vi "Save Correction.vi"() -> ()   [LabVIEW 2017]
uses:
  Globals.vi
panel:
  out "Boolean":bool=TRUE
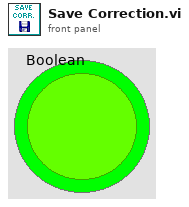
[diagram p1: front panel]
types:
  T1 = cluster{"x shift":dbl, "y shift":dbl, "z shift":dbl, "Theta x":dbl, "Theta y":dbl}
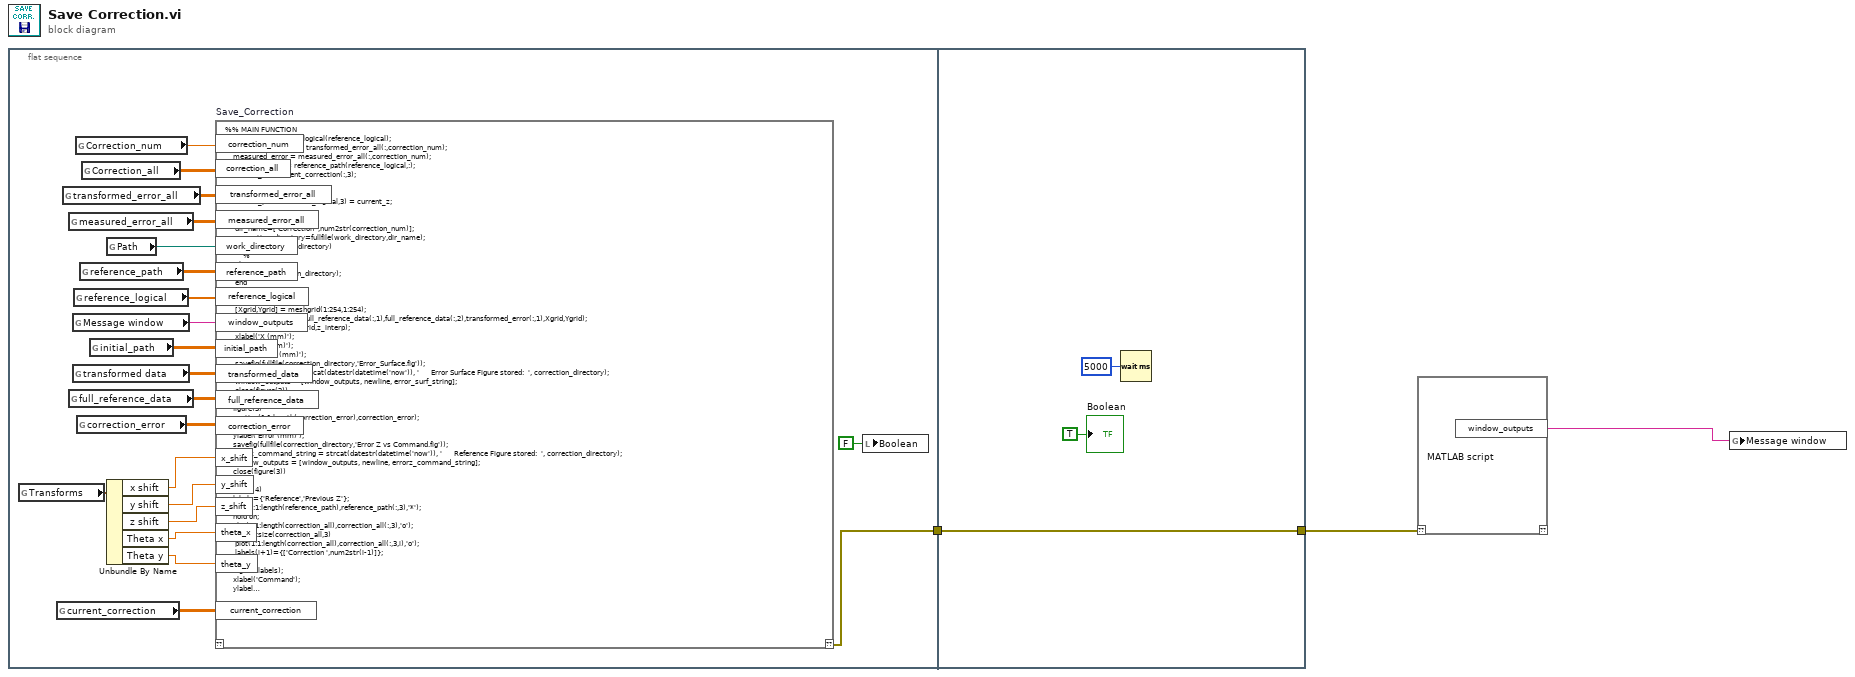
[diagram p0: block diagram]
diagram:
  n1 = flat-sequence {
    tunnel: [w5] -> w1
    tunnel: [w27] -> w2
    tunnel: w1 -> [w27]
    frame #0 {
      n2 = global read "Globals.vi" "Transforms"() -> (w12:T1)
      n3 = global read "Globals.vi" "current_correction"() -> (w6:dbl[][])
      n4 = global read "Globals.vi" "transformed_error_all"() -> (w15:dbl[][])
      n5 = global read "Globals.vi" "measured_error_all"() -> (w16:dbl[][])
      n6 = global read "Globals.vi" "full_reference_data"() -> (w23:dbl[][])
      n7 = global read "Globals.vi" "Message window"() -> (w20:string)
      n8 = global read "Globals.vi" "transformed data"() -> (w22:dbl[][])
      n9 = global read "Globals.vi" "reference_logical"() -> (w19:dbl[])
      n10 = global read "Globals.vi" "Correction_num"() -> (w13:dbl)
      n11 = global read "Globals.vi" "correction_error"() -> (w24:dbl[][])
      n12 = global read "Globals.vi" "reference_path"() -> (w18:dbl[][])
      n13 = global read "Globals.vi" "Correction_all"() -> (w14:dbl[][])
      n14 = global read "Globals.vi" "initial_path"() -> (w21:dbl[][])
      n15 = global read "Globals.vi" "Path"() -> (w17:path)
      n16 = Unbundle By Name(w12) -> ("x shift"=w11:dbl, "y shift"=w10:dbl, "z shift"=w9:dbl, "Theta x"=w8:dbl, "Theta y"=w7:dbl)
      n17 = script code="%% MAIN FUNCTION\n    reference_logical=~logical(reference_logical);\n    transformed_error = transformed_error_all(:,correction_num);\n    measured_error = measured_error_all(:,correction_num);\n    reference_data = reference_path(reference_logical,:);\n    current_z = current_correction(:,3);\n    \n    current_path = initial_path;\n    current_path(reference_logical,3) = current_z;     \n    \n    %%% PLOT ERROR\n     dir_name=['Correction ',num2str(correction_num)];\n     correction_directory=fullfile(work_directory,dir_name);\n     if isdir(correction_directory)\n         %\n     else\n         mkdir(correction_directory);\n     end\n \n     figure(2)\n     [Xgrid,Ygrid] = meshgrid(1:254,1:254);\n     z_interp = griddata(full_reference_data(:,1),full_reference_data(:,2),transformed_error(:,1),Xgrid,Ygrid);\n     zsurf = surf(Xgrid,Ygrid,z_interp);\n     xlabel('X (mm)');\n     ylabel('Y (mm)');\n     zlabel('Error (mm)');\n     savefig(fullfile(correction_directory,'Error_Surface.fig'));\n     error_surf_string = strcat(datestr(datetime('now')), '      Error Surface Figure stored:  ', correction_directory);\n     window_outputs = [window_outputs, newline, error_surf_string];\n     close(figure(2))\n\n    figure(3)\n    scatter(1:1:length(correction_error),correction_error);\n    xlabel('Command');\n    ylabel('Error (mm)');\n    savefig(fullfile(correction_directory,'Error Z vs Command.fig'));\n    errorz_command_string = strcat(datestr(datetime('now')), '      Reference Figure stored:  ', correction_directory);\n    window_outputs = [window_outputs, newline, errorz_command_string];\n    close(figure(3))\n\n    figure(4)\n    labels={'Reference','Previous Z'};\n    plot(1:1:length(reference_path),reference_path(:,3),'*');\n    hold on;\n    plot(1:1:length(correction_all),correction_all(:,3),'o');\n    for i=2:size(correction_all,3)\n     plot(1:1:length(correction_all),correction_all(:,3,i),'o');\n     labels(i+1)={['Correction ',num2str(i-1)]};\n    end\n    legend(labels);\n    xlabel('Command');\n    ylabel('Z (mm)');\n    savefig(fullfile(correction_directory,'Correction and Reference vs Command.fig'));\n    correct_command_string = strcat(datestr(datetime('now')), '      Correction/Reference vs Command Figure stored:  ', correction_directory);\n    window_outputs = [window_outputs, newline, correct_command_string];\n    close(figure(4)) \n\n    figure(5)\n    points=zeros(length(current_correction),3);\n    for i=1:length(current_correction)\n        points(i,1)=current_correction(i,1);\n        points(i,2)=current_correction(i,2);\n        points(i,3)=current_correction(i,3);\n    end\n    plot3(points(:,1),points(:,2),points(:,3));\n    savefig(fullfile(correction_directory,'Path.fig'));\n    correct_path_string = strcat(datestr(datetime('now')), '      Corrected Path Figure stored:  ', correction_directory);\n    window_outputs = [window_outputs, newline, correct_path_string];\n    close(figure(5))\n    csvwrite(fullfile(correction_directory,'Corrected_Path.csv'),current_path);\n    correct_path_csv_string = strcat(datestr(datetime('now')), '      Corrected Path CSV stored:  ', correction_directory);\n    window_outputs = [window_outputs, newline, correct_path_csv_string];\n\n    csvwrite(fullfile(correction_directory,'Error.csv'),transformed_error);\n    error_csv_string = strcat(datestr(datetime('now')), '      Error CSV stored:  ', correction_directory);\n    window_outputs = [window_outputs, newline, error_csv_string];\n\n    %%% Create command for robot based on initial_path\n    oldDir = pwd;\n    cd(function_directory)\n    Module_Output(current_path, correction_directory);\n    cd(oldDir);\n\n    module_string = strcat(datestr(datetime('now')), '      Correction ', num2str(correction_num), ' Module file stored:  ', correction_directory);\n    window_outputs = [window_outputs, newline, module_string];\n\n    % Write Error information to a text file\n    fileID = fopen(fullfile(correction_directory,strcat('Correction ',num2str(correction_num),' Data.txt')),'w');\n    fprintf(fileID,strcat('Correction ',num2str(correction_num)),' Data \\n');\n    fprintf(fileID,'Raw Data Error Magnitude: %4.3f\\n',norm(measured_error));\n    fprintf(fileID,'Transformed Data Error Magnitude: %4.3f\\n',norm(transformed_error));\n    fclose(fileID);\n    correctioninfo_string = strcat(datestr(datetime('now')), '      Correction ', num2str(correction_num), ' Information file stored:  ', correction_directory);\n    window_outputs = [window_outputs, newline, correctioninfo_string];\n\n    % Save Error gridded data\n    x = 0:254;\n    y = 0:254;\n    [X,Y] = meshgrid(x,y);\n    E = scatteredInterpolant(full_reference_data(:,1),full_reference_data(:,2),transformed_error(:,1));\n    error_grid = E(X,Y);\n    csvwrite(fullfile(correction_directory, 'Reference Z Gridded Data.csv'),error_grid);\n    error_grid_string = strcat(datestr(datetime('now')), '      Error Gridded Data .csv stored:  ', correction_directory);\n    window_outputs = [window_outputs, newline, error_grid_string];\n\n    % Save Transformed gridded data\n    x = 0:254;\n    y = 0:254;\n    [X,Y] = meshgrid(x,y);\n    T = scatteredInterpolant(transformed_data(:,1),transformed_data(:,2),transformed_data(:,3));\n    transformed_data_grid = T(X,Y);\n    csvwrite(fullfile(correction_directory, 'Transformed Gridded Data.csv'),transformed_data_grid);\n    tform_grid_string = strcat(datestr(datetime('now')), '      Transformed Gridded Data .csv stored:  ', correction_directory);\n    window_outputs = [window_outputs, newline, tform_grid_string];\n  \n\n    csvwrite(fullfile(correction_directory, 'Measured Data.csv'),transformed_data);\n    tform_grid_string = strcat(datestr(datetime('now')), '      Measured Data .csv stored:  ', correction_directory);\n    window_outputs = [window_outputs, newline, tform_grid_string];\n\n\n%     % Plot Error Magnitude vs Form\n%     xaxis = 1:correction_num;\n%     labels = { 'Initial Command' } ;\n%     error_norms = [];\n%     for i = 1:correction_num\n%         error_norms(i) = norm(transformed_error_all(:,i));\n%         disp(error_norms(i))\n%         labels(i+1)= { strcat('Correction ', num2str(correction_num)) };\n%     end\n%     scatter(xaxis,error_norms,'o', 'b','filled');\n%     grid on;\n%     set(gca, 'XTick',1:correction_num+1, 'XTickLabel', labels);\n%     title('Error Magnitude vs Iteration');\n%     savefig(fullfile(work_directory,'Error Magnitude vs Iteration Plot.fig'));\n\n    % Write Transformation information to a text file\n    fileID = fopen(fullfile(correction_directory,'Transformation Information.txt'),'w');\n    fprintf(fileID,'Transformation Information \\n');\n    fprintf(fileID,'Translation in x (mm): %4.3f\\n',x_shift);\n    fprintf(fileID,'Translation in y (mm): %4.3f\\n',y_shift);\n    fprintf(fileID,'Translation in z (mm): %4.3f\\n',z_shift);\n    fprintf(fileID,'Theta about x-axis (degrees): %4.3f\\n',theta_x);\n    fprintf(fileID,'Theta about y-axis (degrees): %4.3f\\n',theta_y);\n    fclose(fileID);\n    tran_string = strcat(datestr(datetime('now')), '      Transformation Information .txt file stored:  ', work_directory);\n    window_outputs = [window_outputs, newline, tran_string];\n\n\n    % Print to output window\n    window_outputs = [window_outputs, newline, ' ----------- ', newline];" "Save_Correction"("correction_num"=w13, "correction_all"=w14, "transformed_error_all"=w15, "measured_error_all"=w16, "work_directory"=w17, "reference_path"=w18, "reference_logical"=w19, "window_outputs"=w20, "initial_path"=w21, "transformed_data"=w22, "full_reference_data"=w23, "correction_error"=w24, "x_shift"=w11, "y_shift"=w10, "z_shift"=w9, "theta_x"=w8, "theta_y"=w7, "current_correction"=w6) -> ("??"=w5:errorcluster)  [unwired: 1 in]
      n18 = local write "Boolean"(FALSE ("Boolean")) -> ()
    }
    frame #1 {
      n19 = Wait (ms)(milliseconds to wait=u32 5000) -> ()  [unwired: 1 out]
      "Boolean" <- TRUE
    }
  }
  n20 = script code="MATLAB script"("??"=w2) -> ("window_outputs"=w3:string)  [unwired: 1 out]
  n21 = global write "Globals.vi" "Message window"(w3) -> ()
